vi "Basic Level Triggering of Waveforms.vi"() -> ()   [LabVIEW 2020]
doc: "Demonstrates how you can monitor an input signal for trigger conditions. You can specify the trigger condition in terms of hysteresis, slope (rising or falling edge) and level. This example uses cursors to show the different trigger points."
uses:
  <vilib>/measure/mamon.llb/Trigger Detection for N Channel.vi
  <vilib>/measure/NI_MABase.lvlib
  <vilib>/measure/NI_MAPro.lvlib
panel:
  in  "slope":u16[](array[ring])=[1, 1] items=["Falling Edge", "Rising Edge"]
  out "trigger detected?":bool[](array[boolean])
  in  "Stop":bool
  in  "hysteresis":dbl[](array[numeric])=[0.0, 0.0] format="%#.6g"
  in  "level":dbl[](array[numeric])=[0.4, 0.5] format="%#.6g"
  out "Waveform Graph":waveform(dbl)[](graph)
  # "Overview: Demonstrates how to monitor an input signal for trigger conditions. \nRequirements: LabVIEW Full Development System\nInstructions: \n1. Run the VI.  \n2. Change the level, slope, and hysteresis trigger conditions for each of the 2 channels.\n3. Observe that the cursors show each trigger point.\n4. Click Stop to stop the VI."
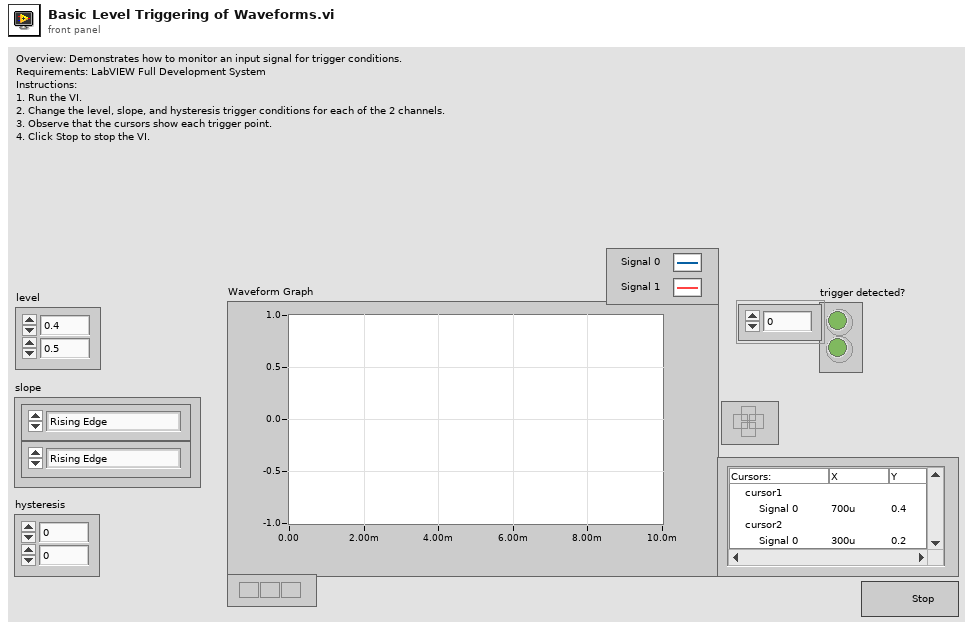
[diagram p1: front panel]
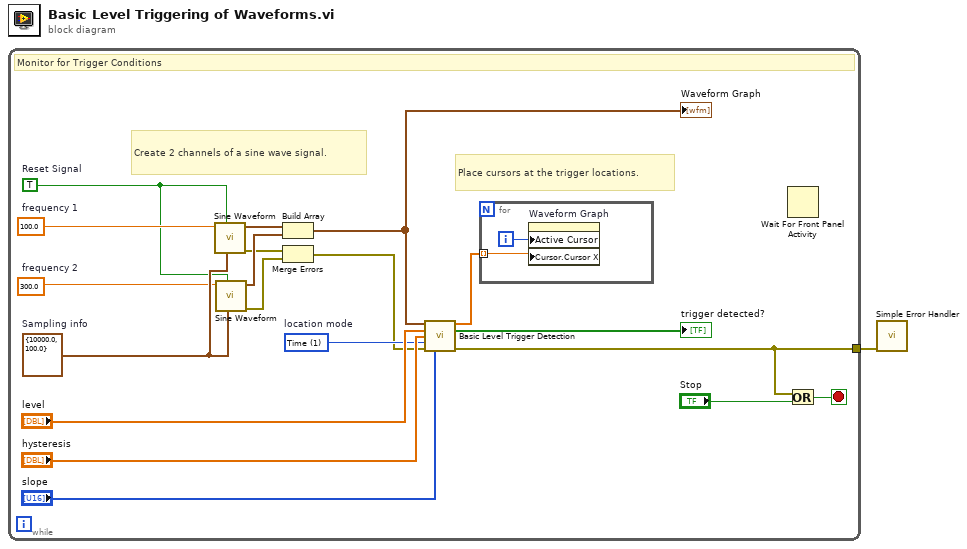
[diagram p0: block diagram]
diagram:
  n1 = while {
    tunnel: [w5] -> w1
    stop <- w8 stop-if-true
    w6 = u16 1 items=["Index", "Time"]  # location mode
    w15 = TRUE  # Reset Signal
    w18 = 300.0  # frequency 2
    w19 = 100.0  # frequency 1
    w20 = cluster{"Fs":dbl, "#s":dbl} {"Fs"=10000.0, "#s"=100.0}  # Sampling info
    # "Create 2 channels of a sine wave signal."
    # "Place cursors at the trigger locations."
    # "Monitor for Trigger Conditions"
    n2 = call <vilib>:"Sine Waveform.vi"("sampling info"=w20, "reset signal"=w15, "frequency"=w19) -> ("error out"=w4:errorcluster, "signal out"=w14:waveform(dbl))  [unwired: 7 in]
    n3 = call <vilib>:"Sine Waveform.vi"("sampling info"=w20, "reset signal"=w15, "frequency"=w18) -> ("error out"=w3:errorcluster, "signal out"=w16:waveform(dbl))  [unwired: 7 in]
    n4 = Build Array(w14, w16) -> (w13:waveform(dbl)[])
    "Waveform Graph" <- w13
    n5 = Merge Errors(w4, w3) -> (w2:errorcluster)
    n6 = call-poly <vilib>:"Basic Level Trigger Detection.vi"("signal in"=w13, "level"="level", "hysteresis"="hysteresis", "location mode"=w6, "error in (no error)"=w2, "trigger slope"="slope") -> ("trigger locations"=w12:dbl[], "trigger detected?"=→"trigger detected?":bool[], "error out"=w5:errorcluster)  [unwired: 7 in]
    n7 = for {
      tunnel: w12 -> [w21] mode=indexing
      i -> [w22]
      n8 = property on="Waveform Graph" class="WFGraph (strict)"("Active Cursor"=w22, "Cursor.Cursor X"=w21) -> ()  [unwired: 2 in, 2 out]
    }
    n9 = Wait For Front Panel Activity() -> ()  [unwired: 3 in, 1 out]
    n10 = Or(x=w5, y="Stop") -> (x .or. y?=w8:bool)
  }
  n11 = call <vilib>:"Simple Error Handler.vi"("error in (no error)"=w1) -> ()  [unwired: 4 in, 5 out]
